vi "百分之60.vi"(11 "数值":dbl) -> (3 "数值 2":dbl)   [LabVIEW 2016]
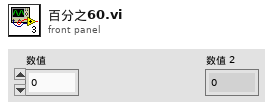
[diagram p1: front panel]
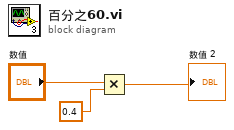
[diagram p0: block diagram]
diagram:
  n1 = Multiply(x="数值", y=0.4) -> (x*y=→"数值 2":dbl)
